vi "__FilterSet_AIDChange.vi"(0 "Param in":cluster{"mode":u8, "AccCode":u32, "AccMask":u32}, 5 "CtrlRef":T1, 7 "EID?":bool, 11 "error in (no error)":errorcluster, 12 "IDRef 2":refnum<vi>[](array[refnum]), 13 "EIDRef 2":refnum<vi>[](array[refnum])) -> (4 "Param out":cluster{"mode":u8, "AccCode":u32, "AccMask":u32}, 15 "error out":errorcluster)   [LabVIEW 2011]
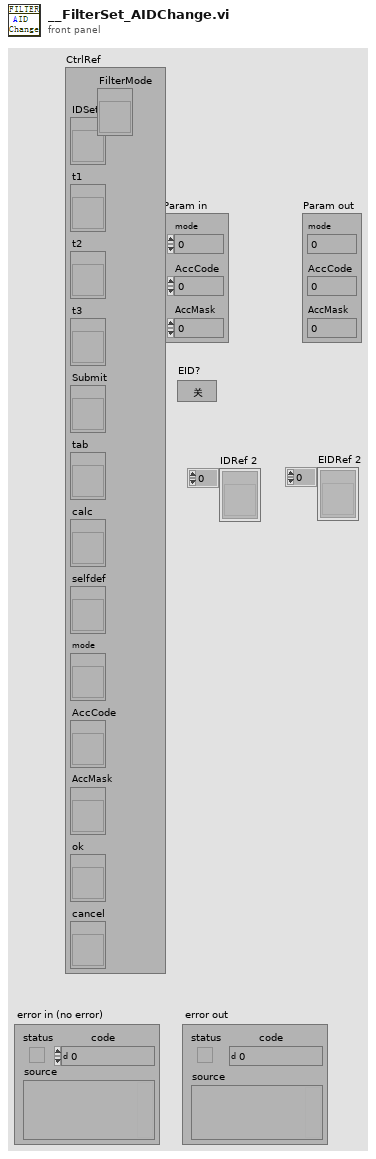
[diagram p1: front panel]
types:
  T1 = cluster{"FilterMode":refnum<vi>, "IDSet":refnum<vi>, "t1":refnum<vi>, "t2":refnum<vi>, "t3":refnum<vi>, "Submit":refnum<vi>, "tab":refnum<vi>, "calc":refnum<vi>, "selfdef":refnum<vi>, "mode":refnum<vi>, "AccCode":refnum<vi>, "AccMask":refnum<vi>, "ok":refnum<vi>, "cancel":refnum<vi>}
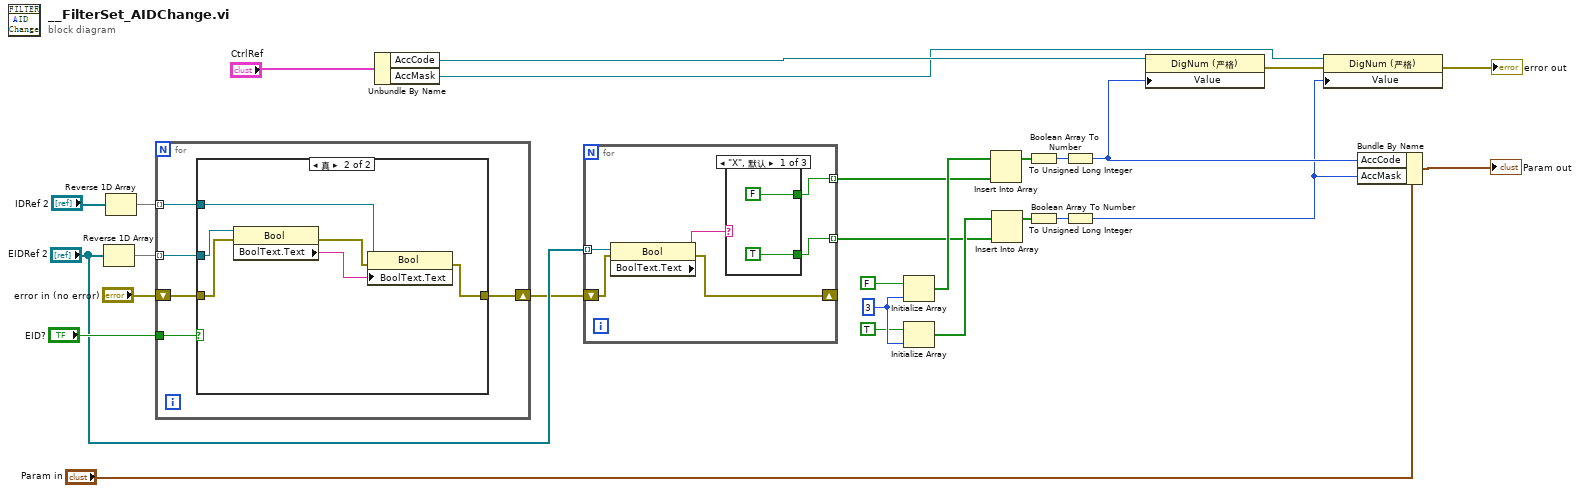
[diagram p0: block diagram]
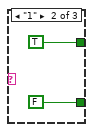
[diagram p2: hidden frame]
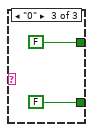
[diagram p3: hidden frame]
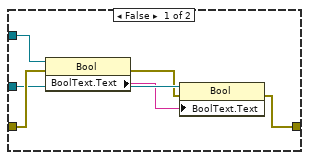
[diagram p4: hidden frame]
diagram:
  w26 = 3 ("维数大小")
  n1 = Reverse 1D Array(array="EIDRef 2") -> (reversed array=w7:refnum<vi>[])
  n2 = Reverse 1D Array(array="IDRef 2") -> (reversed array=w6:refnum<vi>[])
  n3 = for {
    tunnel: w7 -> [w30] mode=indexing
    tunnel: w6 -> [w31] mode=indexing
    shift-right: [w28] -> w3
    shift-left: "error in (no error)" -> [w29]
    tunnel: "EID?" -> [w32]
    n4 = case shown="真" w32 {
      tunnel: w31 -> [w38 w39]
      tunnel: w30 -> [w36 w40]
      tunnel: w29 -> [w37 w44]
      tunnel: [w33 w41] -> w28
      frame False {
        n5 = property class="Bool"(reference=w38, error in=w37) -> (error out=w34:errorcluster, "BoolText.Text"=w35:string)  [unwired: 1 out]
        n6 = property class="Bool"(reference=w36, error in=w34, "BoolText.Text"=w35) -> (error out=w33:errorcluster)  [unwired: 1 out]
      }
      frame True {
        n7 = property class="Bool"(reference=w40, error in=w44) -> (error out=w42:errorcluster, "BoolText.Text"=w43:string)  [unwired: 1 out]
        n8 = property class="Bool"(reference=w39, error in=w42, "BoolText.Text"=w43) -> (error out=w41:errorcluster)  [unwired: 1 out]
      }
    }
  }
  n9 = Unbundle By Name("CtrlRef") -> ("AccCode"=w18:refnum<vi>, "AccMask"=w16:refnum<vi>)
  n10 = for {
    tunnel: "EIDRef 2" -> [w50] mode=indexing
    shift-right: [w48] -> _
    shift-left: w3 -> [w49]
    tunnel: [w46] -> w2 mode=indexing
    tunnel: [w45] -> w1 mode=indexing
    n11 = property class="Bool"(reference=w50, error in=w49) -> (error out=w48:errorcluster, "BoolText.Text"=w47:string)  [unwired: 1 out]
    n12 = case shown="\"X\", 默认" w47 {
      tunnel: [FALSE TRUE FALSE] -> w46
      tunnel: [TRUE FALSE FALSE] -> w45
      frame "X", Default {
      }
      frame "1" {
      }
      frame "0" {
      }
    }
  }
  n13 = Initialize Array(FALSE, w26) -> (w24:bool[])
  n14 = Initialize Array(TRUE, w26) -> (w23:bool[])
  n15 = Insert Into Array(array=w24, new element=w2) -> (w22:bool[])  [unwired: 1 in]
  n16 = Insert Into Array(array=w23, new element=w1) -> (w21:bool[])  [unwired: 1 in]
  n17 = Boolean Array To Number(Boolean array=w22) -> (number=w20:u32)
  n18 = Boolean Array To Number(Boolean array=w21) -> (number=w19:u32)
  n19 = To Unsigned Long Integer(number=w20) -> (unsigned 32bit integer=w13:u32)
  n20 = To Unsigned Long Integer(number=w19) -> (unsigned 32bit integer=w12:u32)
  n21 = property class="DigNum (严格)"(reference=w18, "Value"=w13) -> (error out=w17:errorcluster)  [unwired: 1 in, 1 out]
  n22 = property class="DigNum (严格)"(reference=w16, error in=w17, "Value"=w12) -> (error out=→"error out":errorcluster)  [unwired: 1 out]
  n23 = Bundle By Name(cluster="Param in", "AccCode"=w13, "AccMask"=w12) -> (→"Param out":cluster{"mode":u8, "AccCode":u32, "AccMask":u32})
